vi "GetHits.vi"(8 "duration (pts)":dbl, 9 "Array in":dbl[](array[numeric]), 11 "data":waveform(dbl)[](array[waveform])) -> (3 "Array":cluster{"data":waveform(dbl)[]}[](array[cluster]))   [LabVIEW 2022 SP3]
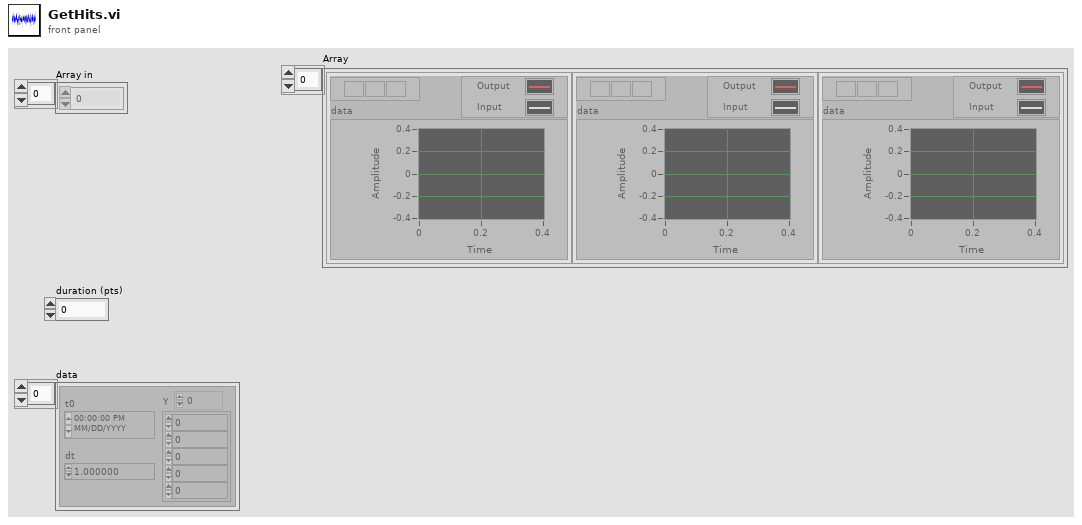
[diagram p1: front panel]
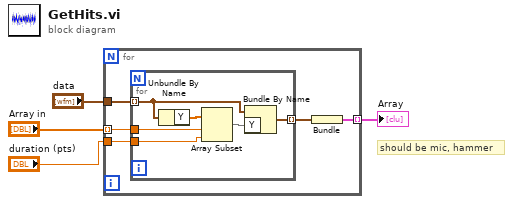
[diagram p0: block diagram]
diagram:
  # "should be mic, hammer"
  n1 = for {
    tunnel: "Array in" -> [w9] mode=indexing
    tunnel: "data" -> [w8]
    tunnel: "duration (pts)" -> [w7]
    tunnel: [w5] -> w4 mode=indexing
    n2 = for {
      tunnel: w9 -> [w15]
      tunnel: w8 -> [w12] mode=indexing
      tunnel: w7 -> [w14]
      tunnel: [w10] -> w6 mode=indexing
      n3 = Unbundle By Name(w12) -> ("Y"=w13:dbl[])
      n4 = Array Subset(array=w13, index=w15, length=w14) -> (w11:dbl[])
      n5 = Bundle By Name(cluster=w12, "Y"=w11) -> (w10:waveform(dbl))
    }
    n6 = Bundle(w6) -> (w5:cluster{waveform(dbl)[]})  [unwired: 1 in]
  }
  "Array" <- w4
